vi "Laser Control.vi"() -> ()   [LabVIEW 2015]
uses:
  <vilib>/Instr/_visa.llb/VISA Configure Serial Port (Instr).vi
panel:
  in  "640 Power (mw)":dbl min=0.0 max=100.0 step=1.0 format="%.1f"
  in  "561 Power (mw)":dbl min=0.0 max=150.0 step=1.0 format="%.1f"
  in  "stop":bool
  in  "640 ON":bool
  in  "561 ON":bool
  in  "488 ON":bool
  # "OFF"
  # "OFF"
  # "OFF"
  # "488 power controled by knob under monitors"
  # "If a laser is greyed out, check the\nconnection or try restarting!"
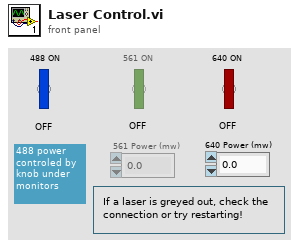
[diagram p1: front panel]
types:
  T1 = enum8{"Enabled", "Disabled", "Disabled and Grayed Out"}
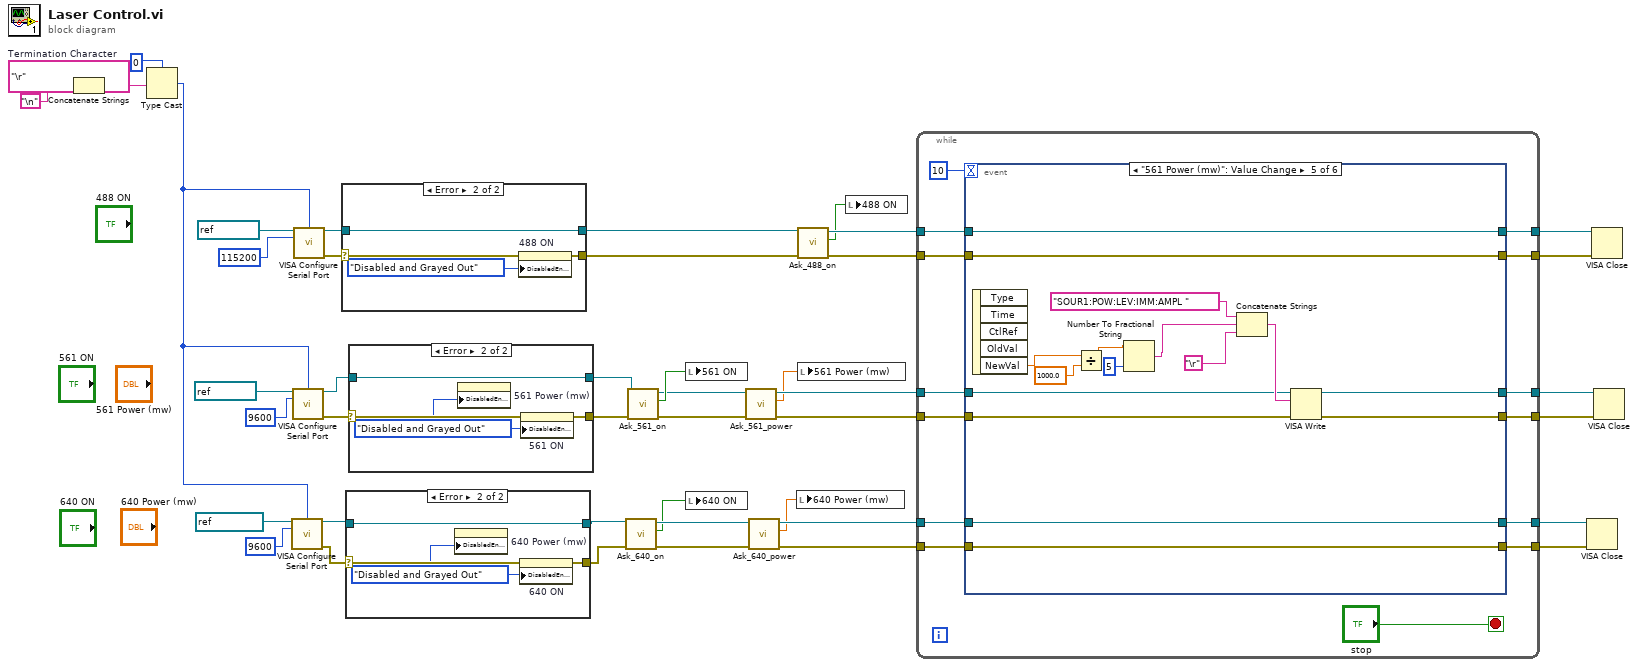
[diagram p0: block diagram]
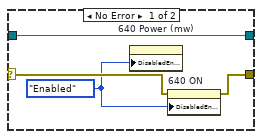
[diagram p2: hidden frame]
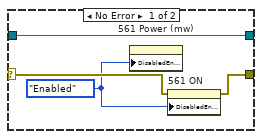
[diagram p3: hidden frame]
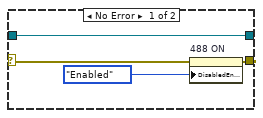
[diagram p4: hidden frame]
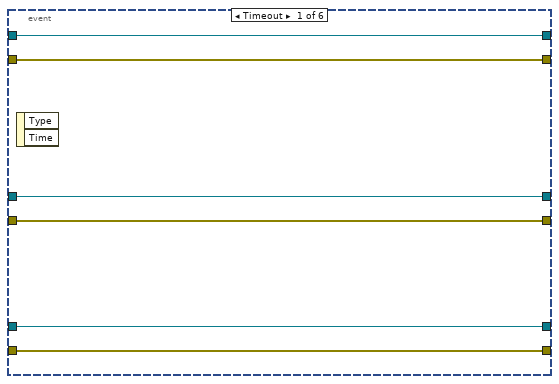
[diagram p5: hidden frame]
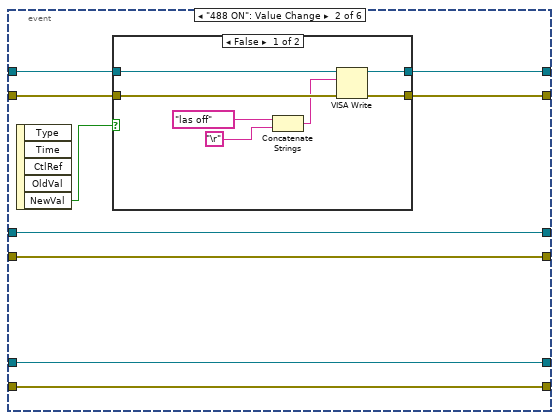
[diagram p6: hidden frame]
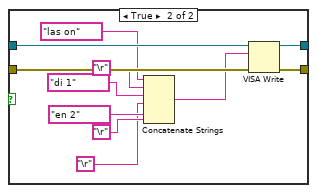
[diagram p7: hidden frame]
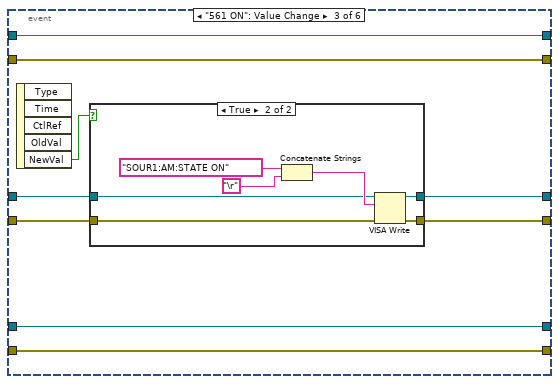
[diagram p8: hidden frame]
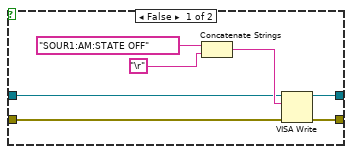
[diagram p9: hidden frame]
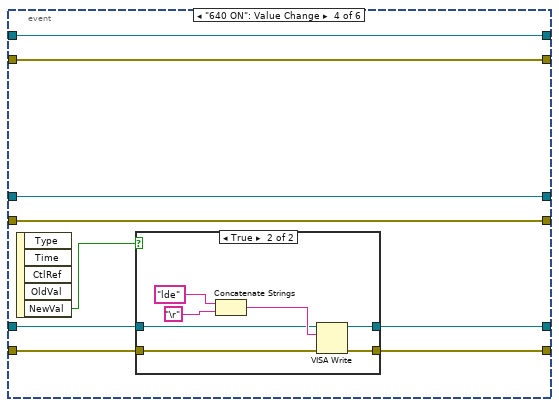
[diagram p10: hidden frame]
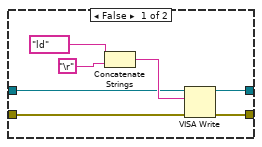
[diagram p11: hidden frame]
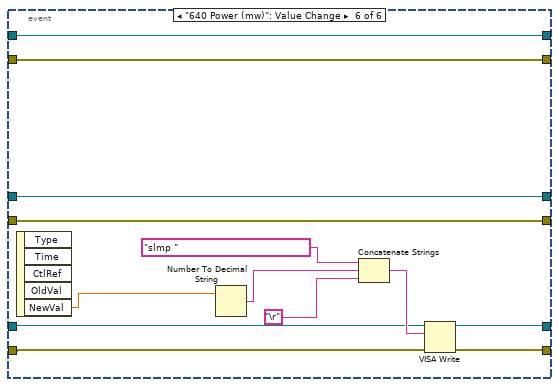
[diagram p12: hidden frame]
diagram:
  w39 = "\r"  # Termination Character
  n1 = Concatenate Strings(w39, "\n") -> (w37:string)
  n2 = Type Cast(type=u8 0, x=w37) -> (*(type *) &x=w29:u8)
  n3 = call-poly "VISA Configure Serial Port"("VISA resource name"=refnum<visa-resource-name> "COM10", "termination char\n(0xA = '\\n' = LF)"=w29, "baud rate (9600)"=u32 9600) -> ("VISA resource name out"=w3:refnum<visa-resource-name>, "error out"=w4:errorcluster)  [unwired: 11 in]
  n4 = call-poly "VISA Configure Serial Port"("VISA resource name"=refnum<visa-resource-name> "COM3", "termination char\n(0xA = '\\n' = LF)"=w29, "baud rate (9600)"=u32 9600) -> ("VISA resource name out"=w8:refnum<visa-resource-name>, "error out"=w6:errorcluster)  [unwired: 11 in]
  n5 = call-poly "VISA Configure Serial Port"("VISA resource name"=refnum<visa-resource-name> "COM1", "termination char\n(0xA = '\\n' = LF)"=w29, "baud rate (9600)"=u32 115200) -> ("VISA resource name out"=w10:refnum<visa-resource-name>, "error out"=w12:errorcluster)  [unwired: 11 in]
  n6 = case shown="Error" w12 {
    selector: w12 -> [w47 w51]
    tunnel: [w46 w52] -> w11
    tunnel: w10 -> [w45 w49]
    tunnel: [w45 w49] -> w9
    frame No Error {
      n7 = property on="488 ON" class="Bool (strict)"(error in=w47, "DisabledEnum"=T1."Enabled" ("Disabled")) -> (error out=w46:errorcluster)  [unwired: 1 in, 1 out]
    }
    frame Error {
      n8 = property on="488 ON" class="Bool (strict)"(error in=w51, "DisabledEnum"=T1."Disabled and Grayed Out" ("Disabled")) -> (error out=w52:errorcluster)  [unwired: 1 in, 1 out]
    }
  }
  n9 = case shown="Error" w4 {
    selector: w4 -> [w56 w59]
    tunnel: [w55 w60] -> w2
    tunnel: w3 -> [w54 w57]
    tunnel: [w54 w57] -> w1
    frame No Error {
      w53 = T1."Enabled" ("Disabled")
      n10 = property on="640 Power (mw)" class="DigNum (strict)"("DisabledEnum"=w53) -> ()  [unwired: 2 in, 2 out]
      n11 = property on="640 ON" class="Bool (strict)"(error in=w56, "DisabledEnum"=w53) -> (error out=w55:errorcluster)  [unwired: 1 in, 1 out]
    }
    frame Error {
      w58 = T1."Disabled and Grayed Out" ("Disabled")
      n12 = property on="640 Power (mw)" class="DigNum (strict)"("DisabledEnum"=w58) -> ()  [unwired: 2 in, 2 out]
      n13 = property on="640 ON" class="Bool (strict)"(error in=w59, "DisabledEnum"=w58) -> (error out=w60:errorcluster)  [unwired: 1 in, 1 out]
    }
  }
  n14 = case shown="Error" w6 {
    selector: w6 -> [w64 w67]
    tunnel: [w63 w68] -> w5
    tunnel: w8 -> [w62 w65]
    tunnel: [w62 w65] -> w7
    frame No Error {
      w61 = T1."Enabled" ("Disabled")
      n15 = property on="561 Power (mw)" class="DigNum (strict)"("DisabledEnum"=w61) -> ()  [unwired: 2 in, 2 out]
      n16 = property on="561 ON" class="Bool (strict)"(error in=w64, "DisabledEnum"=w61) -> (error out=w63:errorcluster)  [unwired: 1 in, 1 out]
    }
    frame Error {
      w66 = T1."Disabled and Grayed Out" ("Disabled")
      n17 = property on="561 Power (mw)" class="DigNum (strict)"("DisabledEnum"=w66) -> ()  [unwired: 2 in, 2 out]
      n18 = property on="561 ON" class="Bool (strict)"(error in=w67, "DisabledEnum"=w66) -> (error out=w68:errorcluster)  [unwired: 1 in, 1 out]
    }
  }
  n19 = call "Ask_640_on.vi"("error in"=w2, "VISA resource name"=w1) -> ("error out"=w20:errorcluster, "640 On"=w19:bool, "VISA resource name out"=w21:refnum<visa-resource-name>)  [unwired: 7 in]
  n20 = call "Ask_561_on.vi"("error in"=w5, "VISA resource name"=w7) -> ("error out"=w17:errorcluster, "561 On"=w18:bool, "VISA resource name out"=w16:refnum<visa-resource-name>)  [unwired: 7 in]
  n21 = local write "561 ON"(w18) -> ()
  n22 = local write "640 ON"(w19) -> ()
  n23 = call "Ask_561_power.vi"("error in"=w17, "VISA resource name"=w16) -> ("error out"=w26:errorcluster, "561 Power"=w23:dbl, "VISA resource name out"=w27:refnum<visa-resource-name>)  [unwired: 7 in]
  n24 = call "Ask_640_power.vi"("error in"=w20, "VISA resource name"=w21) -> ("error out"=w24:errorcluster, "640 Power"=w22:dbl, "VISA resource name out"=w25:refnum<visa-resource-name>)  [unwired: 7 in]
  n25 = local write "640 Power (mw)"(w22) -> ()
  n26 = call "Ask_488_on.vi"("error in"=w11, "VISA resource name"=w9) -> ("error out"=w14:errorcluster, "488 On"=w13:bool, "VISA resource name out"=w15:refnum<visa-resource-name>)  [unwired: 7 in]
  n27 = local write "561 Power (mw)"(w23) -> ()
  n28 = local write "488 ON"(w13) -> ()
  n29 = while {
    tunnel: w15 -> [w82]
    tunnel: w14 -> [w81]
    tunnel: [w80] -> w42
    tunnel: [w79] -> w41
    tunnel: w27 -> [w76]
    tunnel: w26 -> [w75]
    tunnel: [w74] -> w33
    tunnel: [w73] -> w34
    tunnel: [w72] -> w32
    tunnel: [w71] -> w31
    tunnel: w25 -> [w70]
    tunnel: w24 -> [w69]
    stop <- "stop" stop-if-true
    n30 = event shown="[4] \"561 Power (mw)\": Value Change" {
      selector: _ -> [_ _ _ _ _ _]
      dyn-events: _ -> [_ _ _ _ _ _]
      timeout: 10 -> [_ _ _ _ _ _]
      tunnel: w82 -> [w88 w96 w122 w140 w166 w178]
      tunnel: w81 -> [w87 w95 w121 w141 w165 w179]
      tunnel: [w88 w94 w122 w140 w166 w178] -> w80
      tunnel: [w87 w93 w121 w141 w165 w179] -> w79
      tunnel: w76 -> [w86 w92 w123 w142 w175 w180]
      tunnel: w75 -> [w85 w91 w120 w143 w174 w181]
      tunnel: [w85 w91 w119 w143 w173 w181] -> w74
      tunnel: [w86 w92 w118 w142 w172 w180] -> w73
      tunnel: [w84 w90 w117 w147 w168 w183] -> w72
      tunnel: [w83 w89 w116 w146 w167 w182] -> w71
      tunnel: w70 -> [w84 w90 w117 w145 w168 w185]
      tunnel: w69 -> [w83 w89 w116 w144 w167 w184]
      event Timeout {
        n31 = event-data() -> ()  [unwired: 1 in, 2 out]
      }
      event "488 ON": Value Change {
        n32 = event-data() -> ("NewVal"=w97:bool)  [unwired: 1 in, 4 out]
        n33 = case shown="False" w97 {
          tunnel: w96 -> [w104 w115]
          tunnel: w95 -> [w103 w114]
          tunnel: [w102 w113] -> w94
          tunnel: [w101 w112] -> w93
          frame False {
            n34 = Concatenate Strings("las off" ("write buffer"), "\r") -> (w98:string)
            n35 = VISA Write(VISA resource name=w104, write buffer=w98, error in (no error)=w103) -> (VISA resource name out=w102:refnum<visa-resource-name>, error out=w101:errorcluster)  [unwired: 1 out]
          }
          frame True {
            n36 = Concatenate Strings("las on" ("write buffer"), "\r", "di 1" ("write buffer"), "\r", "en 2" ("write buffer"), "\r") -> (w105:string)
            n37 = VISA Write(VISA resource name=w115, write buffer=w105, error in (no error)=w114) -> (VISA resource name out=w113:refnum<visa-resource-name>, error out=w112:errorcluster)  [unwired: 1 out]
          }
        }
      }
      event "561 ON": Value Change {
        n38 = event-data() -> ("NewVal"=w124:bool)  [unwired: 1 in, 4 out]
        n39 = case shown="True" w124 {
          tunnel: w123 -> [w128 w135]
          tunnel: w120 -> [w127 w134]
          tunnel: [w125 w133] -> w119
          tunnel: [w126 w132] -> w118
          frame False {
            n40 = Concatenate Strings("SOUR1:AM:STATE OFF" ("write buffer"), "\r") -> (w129:string)
            n41 = VISA Write(VISA resource name=w128, write buffer=w129, error in (no error)=w127) -> (VISA resource name out=w126:refnum<visa-resource-name>, error out=w125:errorcluster)  [unwired: 1 out]
          }
          frame True {
            n42 = Concatenate Strings("SOUR1:AM:STATE ON" ("write buffer"), "\r") -> (w136:string)
            n43 = VISA Write(VISA resource name=w135, write buffer=w136, error in (no error)=w134) -> (VISA resource name out=w132:refnum<visa-resource-name>, error out=w133:errorcluster)  [unwired: 1 out]
          }
        }
      }
      event "640 ON": Value Change {
        n44 = event-data() -> ("NewVal"=w139:bool)  [unwired: 1 in, 4 out]
        n45 = case shown="True" w139 {
          tunnel: w145 -> [w151 w158]
          tunnel: w144 -> [w150 w157]
          tunnel: [w148 w156] -> w146
          tunnel: [w149 w155] -> w147
          frame False {
            n46 = Concatenate Strings("ld" ("write buffer"), "\r") -> (w152:string)
            n47 = VISA Write(VISA resource name=w151, write buffer=w152, error in (no error)=w150) -> (VISA resource name out=w149:refnum<visa-resource-name>, error out=w148:errorcluster)  [unwired: 1 out]
          }
          frame True {
            n48 = Concatenate Strings("lde" ("write buffer"), "\r") -> (w159:string)
            n49 = VISA Write(VISA resource name=w158, write buffer=w159, error in (no error)=w157) -> (VISA resource name out=w155:refnum<visa-resource-name>, error out=w156:errorcluster)  [unwired: 1 out]
          }
        }
      }
      event "561 Power (mw)": Value Change {
        n50 = event-data() -> ("NewVal"=w170:dbl)  [unwired: 1 in, 4 out]
        n51 = Divide(x=w170, y=1000.0) -> (x/y=w163:dbl)
        n52 = Number To Fractional String(number=w163, precision (6)=i16 5) -> (F-format string=w164:string)  [unwired: 2 in]
        n53 = Concatenate Strings("SOUR1:POW:LEV:IMM:AMPL " ("write buffer"), w164, "\r") -> (w176:string)
        n54 = VISA Write(VISA resource name=w175, write buffer=w176, error in (no error)=w174) -> (VISA resource name out=w172:refnum<visa-resource-name>, error out=w173:errorcluster)  [unwired: 1 out]
      }
      event "640 Power (mw)": Value Change {
        n55 = event-data() -> ("NewVal"=w186:dbl)  [unwired: 1 in, 4 out]
        n56 = Number To Decimal String(number=w186) -> (decimal integer string=w187:string)  [unwired: 1 in]
        n57 = Concatenate Strings("slmp " ("write buffer"), w187, "\r") -> (w189:string)
        n58 = VISA Write(VISA resource name=w185, write buffer=w189, error in (no error)=w184) -> (VISA resource name out=w183:refnum<visa-resource-name>, error out=w182:errorcluster)  [unwired: 1 out]
      }
    }
  }
  n59 = VISA Close(VISA resource name=w32, error in (no error)=w31) -> ()  [unwired: 1 out]
  n60 = VISA Close(VISA resource name=w42, error in (no error)=w41) -> ()  [unwired: 1 out]
  n61 = VISA Close(VISA resource name=w34, error in (no error)=w33) -> ()  [unwired: 1 out]
